vi "PROCESS_VI.vi"(7 "simulazione":bool, 8 "error in (no error)":errorcluster, 10 "variant":variant, 11 "Queue Name":string) -> (0 "error out":errorcluster, 2 "Stopped":bool)   [LabVIEW 2019]
uses:
  TypeDef/Cluster acquisizioni.ctl
  Globals.vi
panel:
  out "In queue":i32
  out "STATO":string
  out "LOOP TIME (ms)":u32
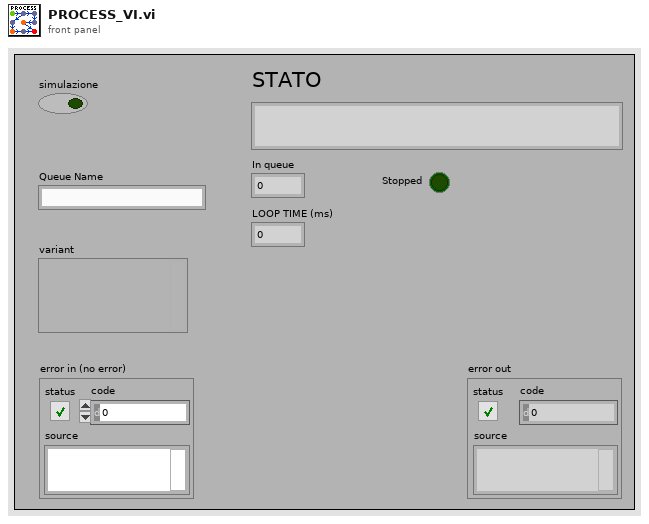
[diagram p1: front panel]
types:
  T1 = cluster{"Array of elements":cluster{"String":string, "variant":variant}[], "Single element":cluster{"String":string, "variant":variant}, "enque at\nopposite end (F)":bool, "no replications (F)":bool}
  T2 = typedef "Cluster acquisizioni.ctl" = cluster{"N°Acq":i16, "Periodo":dbl, "acq in corso":bool, "Acquisizione":bool, "Slide":u8, "Inserisci Acq.":bool}
  T3 = enum32{"Invalid", "Standard", "Closed", "Hidden", "Minimized", "Maximized"}
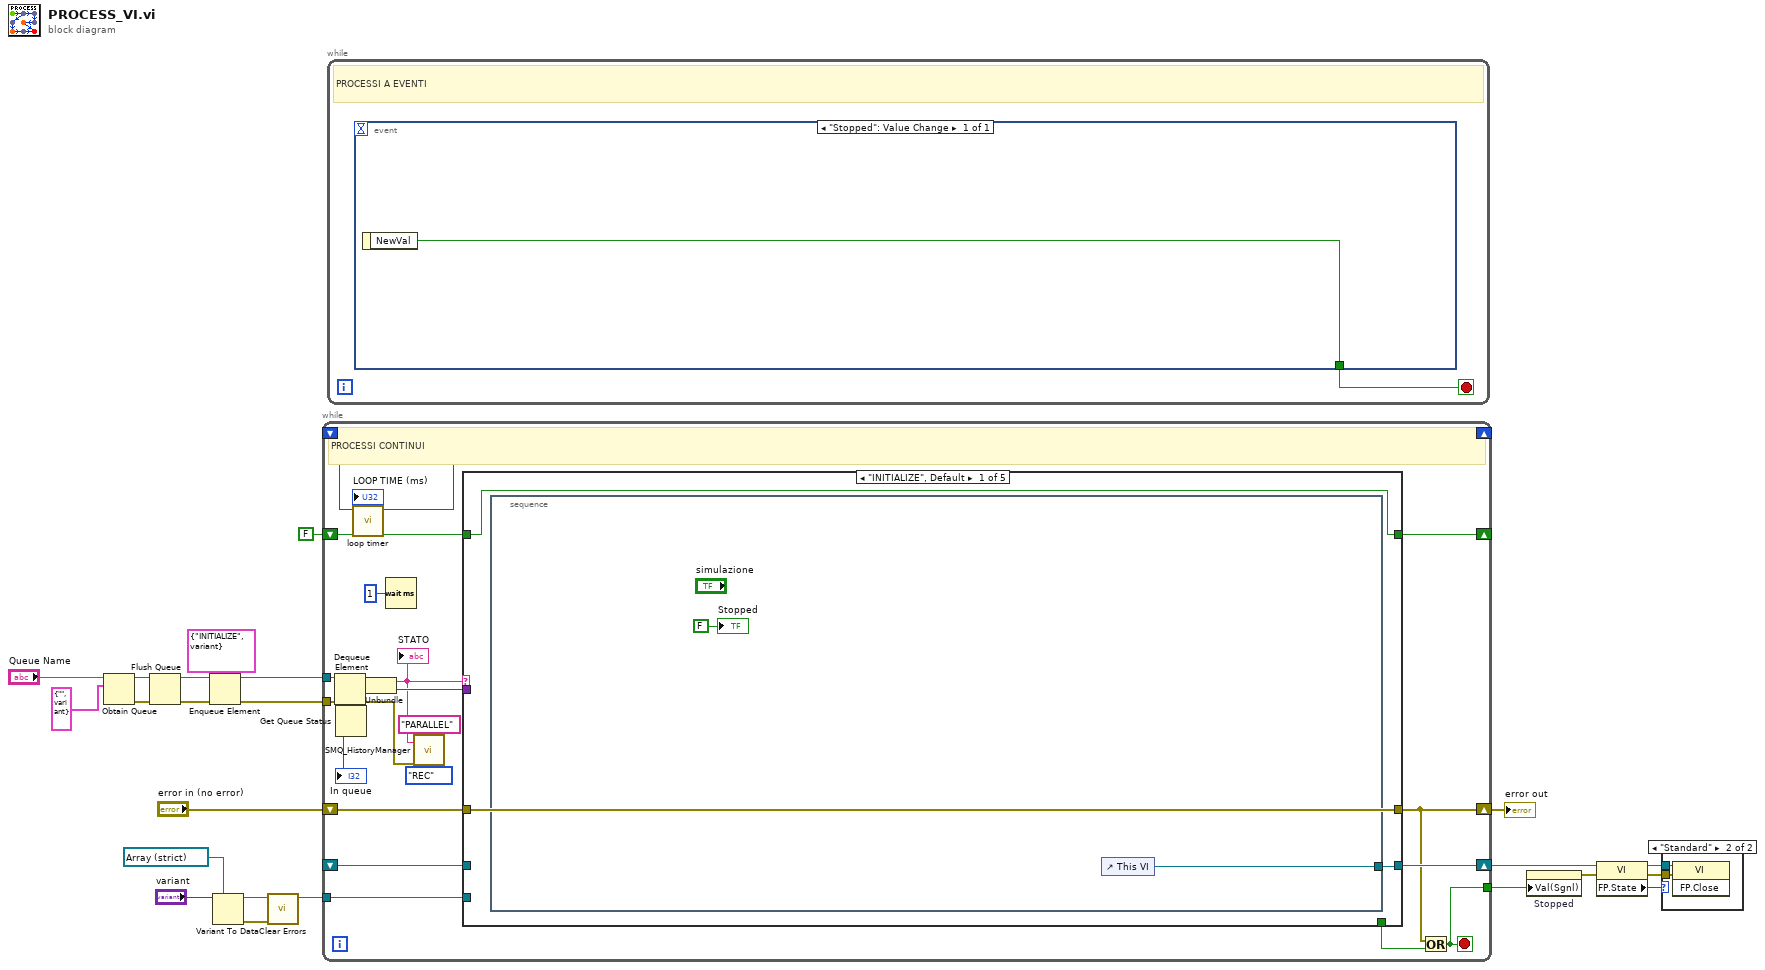
[diagram p0: block diagram]
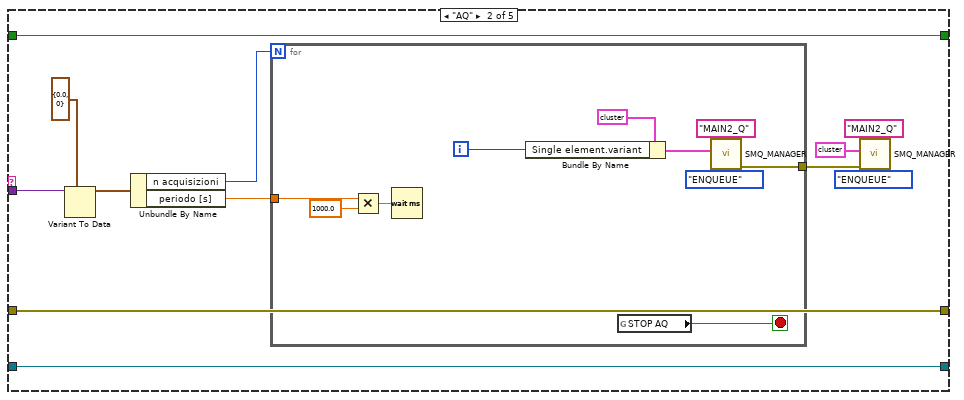
[diagram p3: hidden frame]
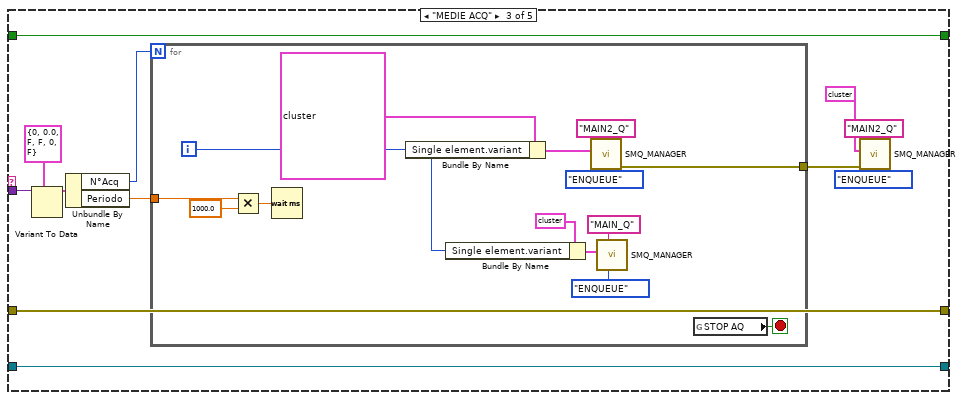
[diagram p4: hidden frame]
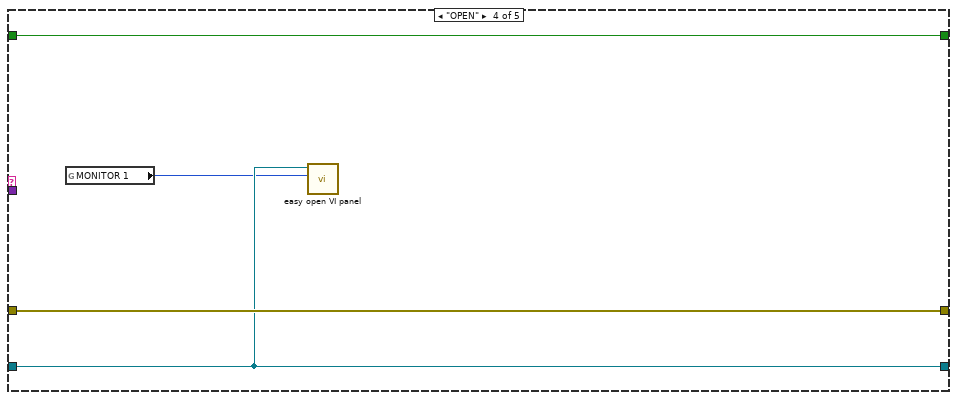
[diagram p5: hidden frame]
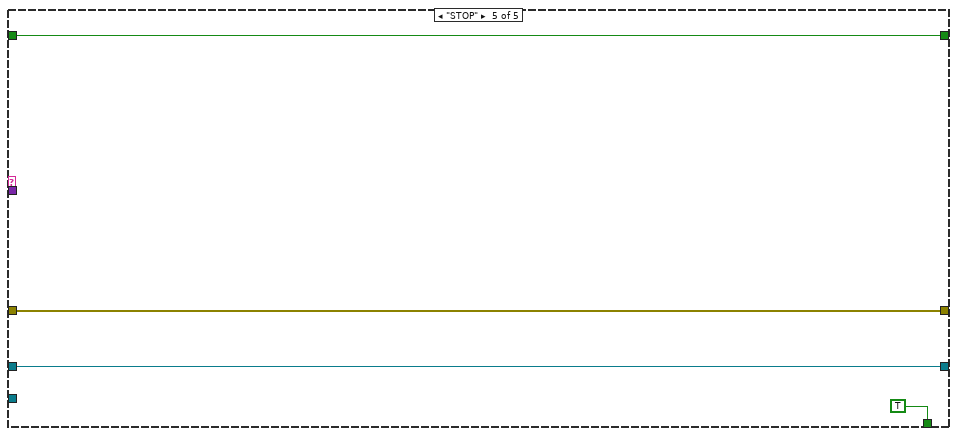
[diagram p6: hidden frame]
diagram:
  n1 = Obtain Queue(name (unnamed)="Queue Name", element data type=cluster{"String":string, "variant":variant} {"String"="", "variant"=variant} ("element")) -> (queue out=w8:refnum<queue>, error out=w7:errorcluster)  [unwired: 3 in, 1 out]
  n2 = Flush Queue(queue=w8, error in (no error)=w7) -> (queue out=w5:refnum<queue>, error out=w4:errorcluster)  [unwired: 1 out]
  n3 = Enqueue Element(queue=w5, element=cluster{"String":string, "variant":variant} {"String"="INITIALIZE", "variant"=variant}, error in (no error)=w4) -> (queue out=w10:refnum<queue>, error out=w9:errorcluster)  [unwired: 1 in, 1 out]
  n4 = Variant To Data(type=refnum<vi> refnum ("TABELLA PUNTI"), Variant="variant") -> (data=w21:refnum<vi>, error out=w2:errorcluster)  [unwired: 1 in]
  n5 = call <vilib>:"Clear Errors.vi"("error in (no error)"=w2) -> ()  [unwired: 5 in, 2 out]
  n6 = while {
    shift-right: [w45] -> _
    shift-left: _ -> [w44]
    shift-right: [w42] -> w13
    shift-left: _ -> [w41]
    shift-right: [w38] -> w16
    shift-left: "error in (no error)" -> [w40]
    tunnel: w21 -> [w37]
    tunnel: w10 -> [w35]
    tunnel: w9 -> [w36]
    tunnel: [w32] -> w18
    shift-right: [w27] -> _
    shift-left: FALSE ("DO") -> [w26]
    stop <- w32 stop-if-true
    # "PROCESSI CONTINUI"
    n7 = Dequeue Element(queue=w35, error in (no error)=w36) -> (queue out=w25:refnum<queue>, element=w34:cluster{"String":string, "variant":variant}, error out=w29:errorcluster)  [unwired: 1 in, 1 out]
    n8 = Get Queue Status(queue=w25) -> (# elements in queue=→"In queue":i32)  [unwired: 2 in, 7 out]
    n9 = call <userlib>:"loop timer.vi"("millisecond timer IN"=w44) -> ("millisecond timer OUT"=w45:u32, "LOOP TIME (ms)"=→"LOOP TIME (ms)":u32)  [unwired: 9 in]
    n10 = Unbundle(w34) -> ("String"=w30:string, "variant"=w33:variant)
    "STATO" <- w30
    n11 = Wait (ms)(milliseconds to wait=u32 1) -> ()  [unwired: 1 out]
    n12 = call <userlib>:"SMQ_HistoryManager.vi"("Caller VI"="PARALLEL", "State"=w30, "error in (no error)"=w29, "Function"=enum16{"INITIALIZE", "REC", "STOP"}."REC") -> ()  [unwired: 14 in, 2 out]
    n13 = case shown="\"INITIALIZE\", Default" w30 {
      tunnel: [_ _ _ _ TRUE] -> w39
      tunnel: [w48 w62 w84 w101 w105] -> w42
      tunnel: w41 -> [_ w62 w84 w101 w105]
      tunnel: w40 -> [w47 w61 w83 w102 w104]
      tunnel: [w47 w61 w83 w102 w104] -> w38
      tunnel: w37 -> [_ _ _ _ _]
      tunnel: w33 -> [_ w59 w81 _ _]
      tunnel: [w46 w60 w82 w100 w103] -> w27
      tunnel: w26 -> [w46 w60 w82 w100 w103]
      frame "INITIALIZE", Default {
        n14 = stacked-sequence {
          tunnel: [w50] -> w48
          frame #0 {
            n15 = control-ref of="This VI"() -> (w50:refnum<vi>)
            "Stopped" <- FALSE ("Stop")
          }
        }
      }
      frame "AQ" {
        n16 = Variant To Data(type=cluster{"periodo [s]":dbl, "n acquisizioni":u8} {"periodo [s]"=0.0, "n acquisizioni"=0} ("Value"), Variant=w59) -> (data=w58:cluster{"periodo [s]":dbl, "n acquisizioni":u8})  [unwired: 1 in, 1 out]
        n17 = Unbundle By Name(w58) -> ("n acquisizioni"=w57:u8, "periodo [s]"=w56:dbl)
        n18 = for {
          N: w57 -> [_]
          tunnel: w56 -> [w72]
          tunnel: [w68] -> w52
          i -> [w69]
          stop <- w67 stop-if-true
          n19 = Multiply(x=w72, y=1000.0) -> (x*y=w70:dbl)
          n20 = Wait (ms)(milliseconds to wait=w70) -> ()  [unwired: 1 out]
          n21 = Bundle By Name(cluster=T1 {"Array of elements"=[], "Single element"={"String"="AQ", "variant"=variant}, "enque at\nopposite end (F)"=FALSE, "no replications (F)"=FALSE} ("Enqueue cluster"), "Single element.variant"=w69) -> (w63:T1)
          n22 = global read "Globals.vi" "STOP AQ"() -> (w67:bool)
          n23 = call <userlib>:"SMQ_MANAGER.vi"("Function"=enum16{"INITIALIZE", "ENQUEUE", "STOP ALL"}."ENQUEUE", "Queue name"="MAIN2_Q", "Enqueue cluster"=w63) -> ("error out"=w68:errorcluster)  [unwired: 8 in]
        }
        n24 = call <userlib>:"SMQ_MANAGER.vi"("Function"=enum16{"INITIALIZE", "ENQUEUE", "STOP ALL"}."ENQUEUE", "Queue name"="MAIN2_Q", "error in (no error)"=w52, "Enqueue cluster"=T1 {"Array of elements"=[], "Single element"={"String"="CALCOLO INCERTEZZA", "variant"=variant}, "enque at\nopposite end (F)"=FALSE, "no replications (F)"=FALSE}) -> ()  [unwired: 7 in, 1 out]
      }
      frame "MEDIE ACQ" {
        n25 = Variant To Data(type=T2 {"N°Acq"=0, "Periodo"=0.0, "acq in corso"=FALSE, "Acquisizione"=FALSE, "Slide"=0, "Inserisci Acq."=FALSE} ("Value"), Variant=w81) -> (data=w80:T2)  [unwired: 1 in, 1 out]
        n26 = Unbundle By Name(w80) -> ("N°Acq"=w79:i16, "Periodo"=w78:dbl)
        n27 = for {
          N: w79 -> [_]
          tunnel: w78 -> [w98]
          tunnel: [w95] -> w74
          i -> [w85]
          stop <- w94 stop-if-true
          n28 = Multiply(x=w98, y=1000.0) -> (x*y=w96:dbl)
          n29 = Wait (ms)(milliseconds to wait=w96) -> ()  [unwired: 1 out]
          n30 = Bundle By Name(cluster=T1 {"Array of elements"=[], "Single element"={"String"="ACQ PER MEDIE", "variant"=variant}, "enque at\nopposite end (F)"=FALSE, "no replications (F)"=FALSE} ("Enqueue cluster"), "Single element.variant"=w85) -> (w90:T1)
          n31 = Bundle By Name(cluster=T1 {"Array of elements"=[], "Single element"={"String"="AGGIORNA #ACQ", "variant"=variant}, "enque at\nopposite end (F)"=FALSE, "no replications (F)"=FALSE} ("Enqueue cluster"), "Single element.variant"=w85) -> (w89:T1)
          n32 = call <userlib>:"SMQ_MANAGER.vi"("Function"=enum16{"INITIALIZE", "ENQUEUE", "STOP ALL"}."ENQUEUE", "Queue name"="MAIN2_Q", "Enqueue cluster"=w90) -> ("error out"=w95:errorcluster)  [unwired: 8 in]
          n33 = call <userlib>:"SMQ_MANAGER.vi"("Function"=enum16{"INITIALIZE", "ENQUEUE", "STOP ALL"}."ENQUEUE", "Queue name"="MAIN_Q", "Enqueue cluster"=w89) -> ()  [unwired: 8 in, 1 out]
          n34 = global read "Globals.vi" "STOP AQ"() -> (w94:bool)
        }
        n35 = call <userlib>:"SMQ_MANAGER.vi"("Function"=enum16{"INITIALIZE", "ENQUEUE", "STOP ALL"}."ENQUEUE", "Queue name"="MAIN2_Q", "error in (no error)"=w74, "Enqueue cluster"=T1 {"Array of elements"=[], "Single element"={"String"="CALCOLO MEDIE", "variant"=variant}, "enque at\nopposite end (F)"=FALSE, "no replications (F)"=FALSE}) -> ()  [unwired: 7 in, 1 out]
      }
      frame "OPEN" {
        n36 = global read "Globals.vi" "MONITOR 1"() -> (w99:u8)
        n37 = call <userlib>:"easy open VI panel.vi"("Monitor(1)"=w99, "VI in"=w101) -> ()  [unwired: 9 in, 1 out]
      }
      frame "STOP" {
      }
    }
    n38 = Or(x=w38, y=w39) -> (x .or. y?=w32:bool)
  }
  "error out" <- w16
  n39 = while {
    stop <- w107 stop-if-true
    # "PROCESSI A EVENTI"
    n40 = event shown="[0] \"Stopped\": Value Change" {
      selector: _ -> [_]
      dyn-events: _ -> [_]
      timeout: _ -> [_]
      tunnel: [w108] -> w107
      event "Stopped": Value Change {
        n41 = event-data() -> ("NewVal"=w108:bool)  [unwired: 1 in]
      }
    }
  }
  n42 = property on="Stopped" class="Bool (strict)"("Val(Sgnl)"=w18) -> (error out=w12:errorcluster)  [unwired: 2 in, 1 out]
  n43 = property class="VI"(reference=w13, error in=w12) -> (reference out=w15:refnum<vi>, error out=w11:errorcluster, "FP.State"=w14:T3)
  n44 = case shown="\"Standard\"" w14 {
    tunnel: w15 -> [_ w110]
    tunnel: w11 -> [_ w109]
    frame "Invalid", Default {
    }
    frame "Standard" {
      n45 = invoke class="VI" method="FP.Close"(reference=w110, error in=w109) -> ()  [unwired: 1 in, 3 out]
    }
  }
